vi "phd_pect.vi"() -> ()   [LabVIEW 2018]
uses:
  <vilib>/Instr/_visa.llb/VISA Configure Serial Port (Instr).vi
panel:
  out "str_ai_output":string caption="AI Output"
  out "num_sensor_sam_per_cycle":u32 caption="Samples/Cycle"
  in  "cbx_sensor_sam_rate":string(combo) caption="Sample Rate (Hz)"
  in  "num_pulse_samples":u32=3 caption="Samples" max=10000 step=100
  in  "Hidden Controls":T1(tab)
  out "baud rate":u32=115200
  out "timeout_default":u32=100
  out "termination char":u8
  out "timeout_for_small_data":u32=100
  out "CMD_ID_GET":string
  out "CMD_ID_RUN":string
  out "CMD_ID_NONE":string
  out "CMD_ID_SET":string
  out "CMD_RUN_NONE":string
  out "CMD_RUN_START":string
  out "CMD_RUN_STOP":string
  out "PG_PULSE_NONE":string
  out "PG_PULSE_SQUARE":string
  out "PG_PULSE_SINE":string
  out "RESPONSE_LEN":u32=32
  out "TIM_FREQ":u32
  out "has_response":bool=TRUE
  out "ADC_CONVERSION_CYCLES":dbl=8.5
  out "ADC_FREQ":u32=64000000
  out "ADC_SAMPLING_TIME":dbl[](array[numeric])
  out "ADC_CLOCK_PRESCALER":u32[](array[numeric])
  out "sam_rates":cluster{u32, u32, dbl}[](array[cluster])
  out "cbx_sensor_sam_rate_sel_idx":u32
  in  "num_senor_read_samples":u32=3 caption="Read Samples" max=10000 step=100
  in  "num_pulse_min_val":dbl=1.0 caption="Minimum Value (V)" min=0.0 max=1.0 step=0.1
  in  "num_pulse_dutyc":u32=100 caption="Duty Cycle (%)" max=100 step=10
  in  "num_pulse_max_val":dbl=3.3 caption="Maximum Value (V)" min=0.0 max=3.3 step=0.1
  out "write buffer":string
  in  "btn_get":bool
  in  "cbx_pulse_type":string(combo) caption="Type"
  in  "num_pulse_freq":u32=200 caption="Frequency (Hz)" max=2000 step=100
  in  "btn_set":bool
  in  "btn_start_stop":bool
  in  "VISA resource name":refnum<visa-resource-name>
  out "read buffer":string
  out "Waveform Graph":u8[](graph)
  # "Communication"
  # "Settings"
  # "Pulse"
  # "Sensor"
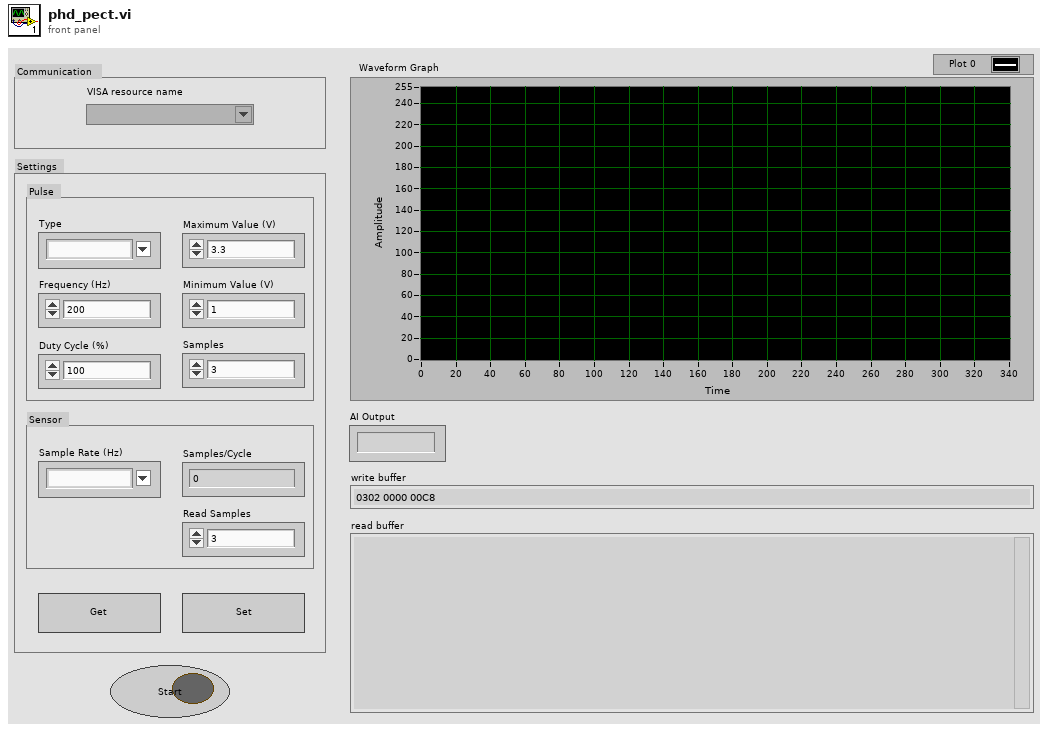
[diagram p1: front panel]
types:
  T1 = enum32{"Page 1", "Page 2", "Page 3", "Page 4", "Page 5"}
  T2 = enum8{"Enabled", "Disabled", "Disabled and Grayed Out"}
  T3 = enum16{"big-endian, network order", "native, host order", "little-endian"}
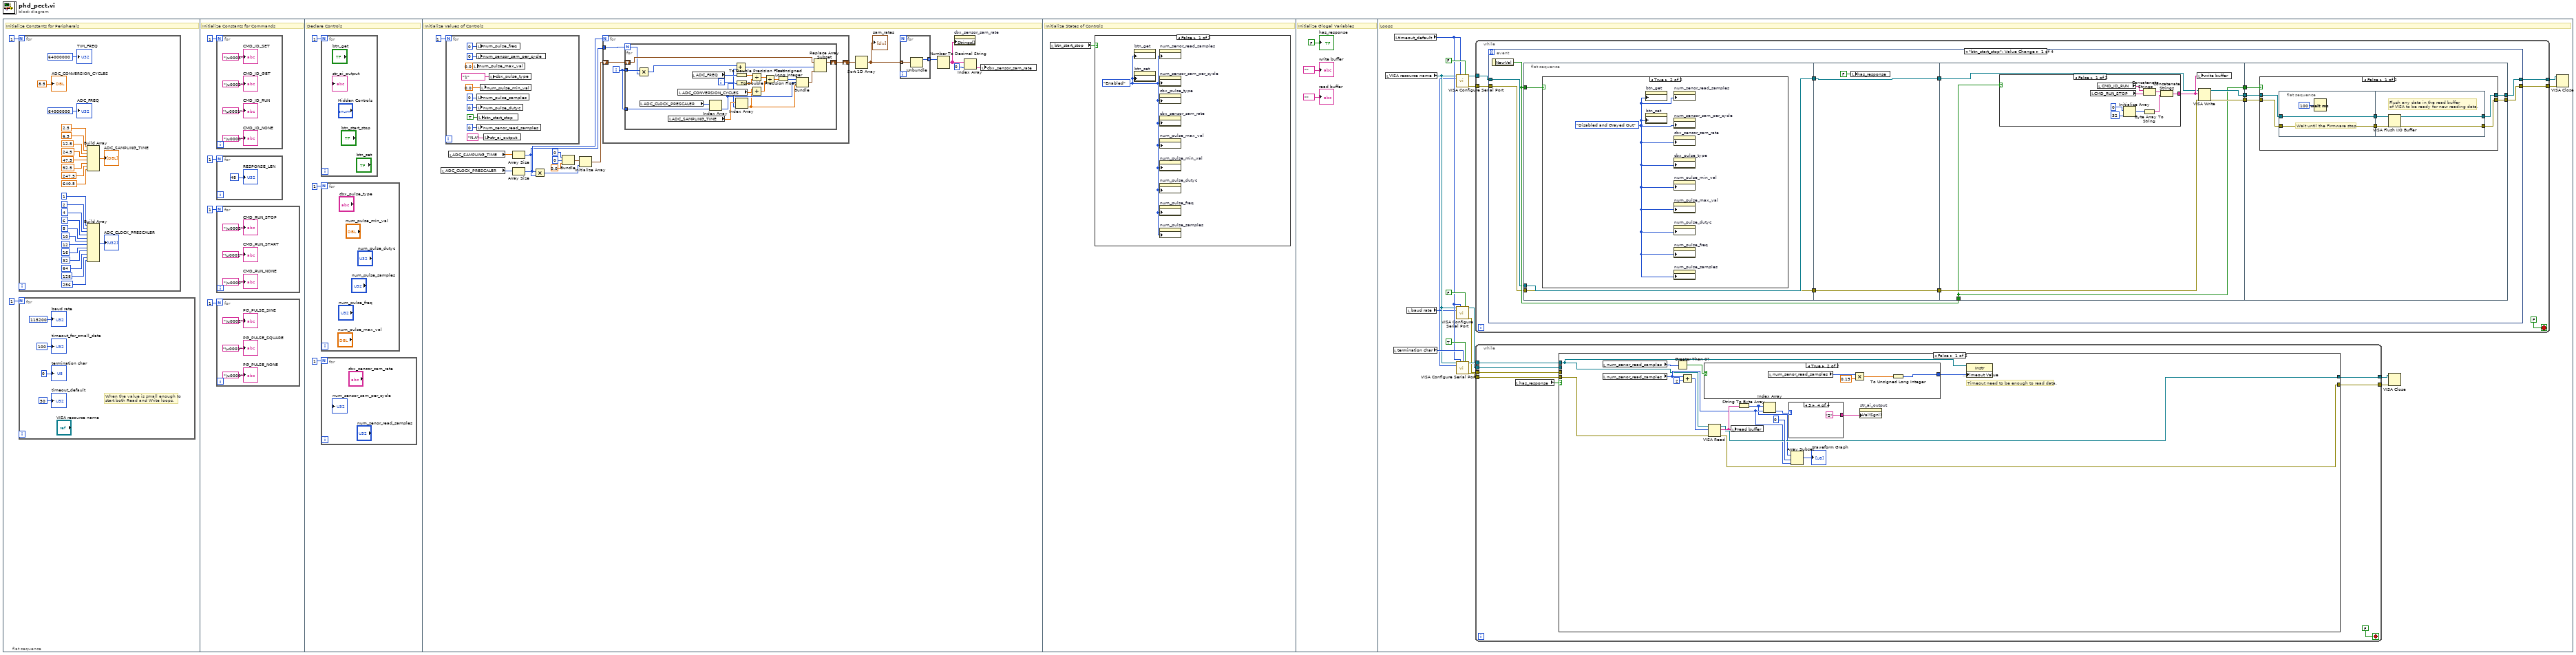
[diagram p0: block diagram]
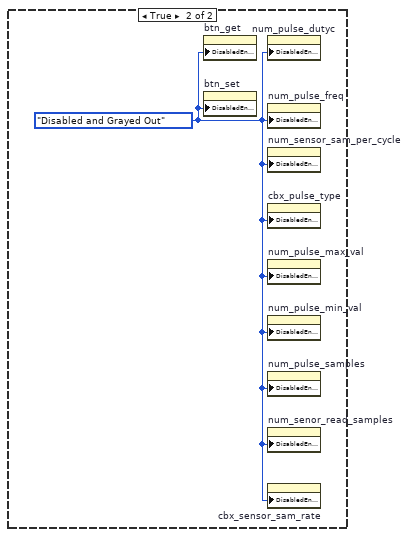
[diagram p2: hidden frame]
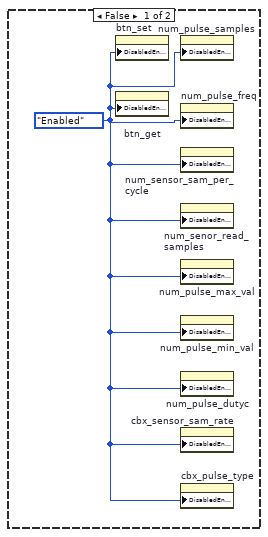
[diagram p3: hidden frame]
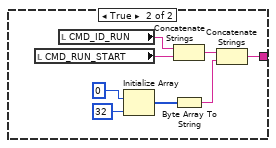
[diagram p4: hidden frame]
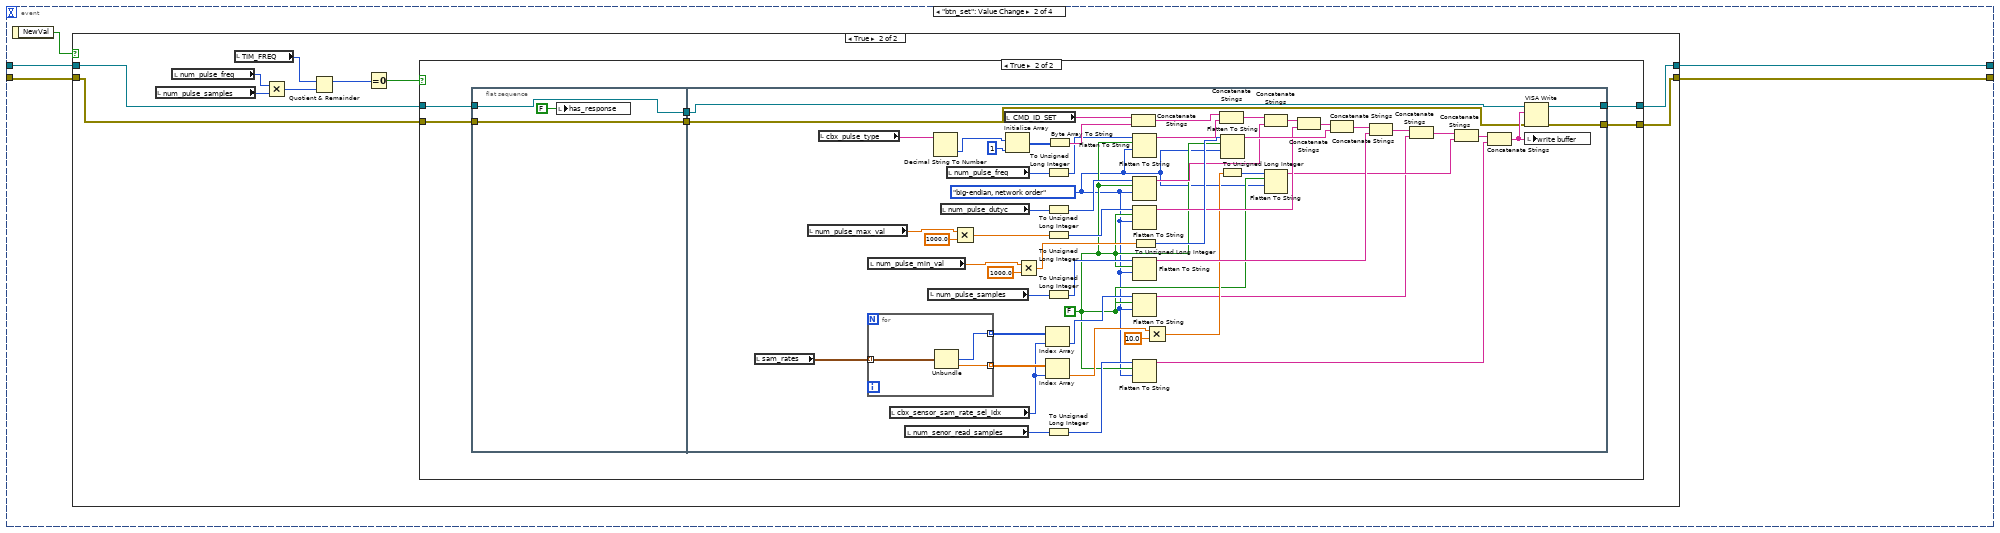
[diagram p6: hidden frame]
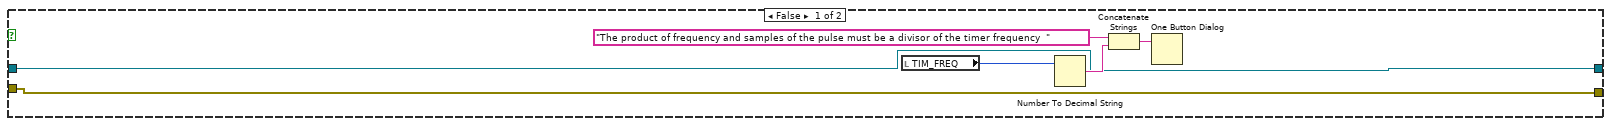
[diagram p8: hidden frame]
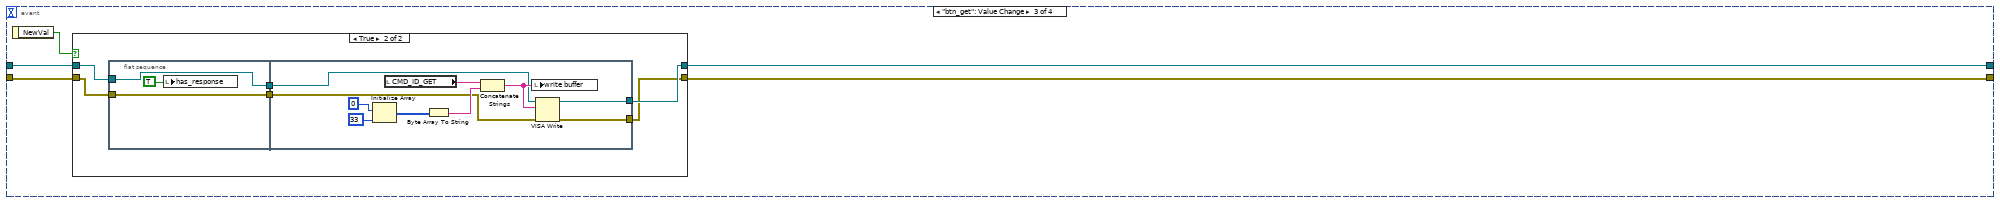
[diagram p9: hidden frame]
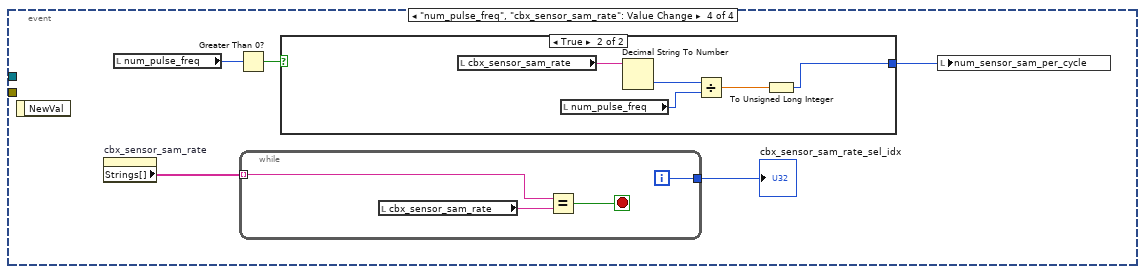
[diagram p11: hidden frame]
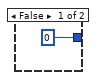
[diagram p12: hidden frame]
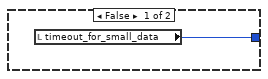
[diagram p13: hidden frame]
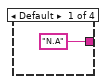
[diagram p14: hidden frame]
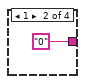
[diagram p15: hidden frame]
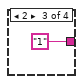
[diagram p16: hidden frame]
diagram:
  n1 = flat-sequence {
    frame #0 {
      # "Initialize Constants for Peripherals"
      n2 = for {
        N: 1 -> [_]
        n3 = Build Array(2.5 ("element"), 6.5 ("element"), 12.5 ("element"), 24.5 ("element"), 47.5 ("element"), 92.5 ("element"), 247.5 ("element"), 640.5 ("element")) -> (→"ADC_SAMPLING_TIME":dbl[])
        n4 = Build Array(u32 1 ("element"), u32 2 ("element"), u32 4 ("element"), u32 6 ("element"), u32 8 ("element"), u32 10 ("element"), u32 12 ("element"), u32 16 ("element"), u32 32 ("element"), u32 64 ("element"), u32 128 ("element"), u32 256 ("element")) -> (→"ADC_CLOCK_PRESCALER":u32[])
        "ADC_CONVERSION_CYCLES" <- 8.5
        "ADC_FREQ" <- 64000000
        "TIM_FREQ" <- 64000000
      }
      n5 = for {
        N: 1 -> [_]
        # "When the value is small enough to\nstart both Read and Write loops."
        "baud rate" <- u32 115200 ("baud rate (9600)")
        "timeout_default" <- u32 50 ("timeout (10sec)")
        "termination char" <- u8 0 ("termination char\n(0xA = '\\n' = LF)")
        "timeout_for_small_data" <- u32 100 ("timeout_default 2")
      }
    }
    frame #1 {
      # "Initialize Constants for Commands"
      n6 = for {
        N: 1 -> [_]
        "CMD_ID_NONE" <- "\u0000"
        "CMD_ID_RUN" <- "\u0001"
        "CMD_ID_GET" <- "\u0002"
        "CMD_ID_SET" <- "\u0003"
      }
      n7 = for {
        N: 1 -> [_]
        "RESPONSE_LEN" <- 48
      }
      n8 = for {
        N: 1 -> [_]
        "CMD_RUN_NONE" <- "\u0000"
        "CMD_RUN_START" <- "\u0001"
        "CMD_RUN_STOP" <- "\u0002"
      }
      n9 = for {
        N: 1 -> [_]
        "PG_PULSE_NONE" <- "\u0000"
        "PG_PULSE_SQUARE" <- "\u0001"
        "PG_PULSE_SINE" <- "\u0002"
      }
    }
    frame #2 {
      # "Declare Controls"
      n10 = for {
        N: 1 -> [_]
      }
      n11 = for {
        N: 1 -> [_]
      }
      n12 = for {
        N: 1 -> [_]
      }
    }
    frame #3 {
      # "Initialize Values of Controls"
      n13 = local read "ADC_CLOCK_PRESCALER"() -> (w60:u32[])
      n14 = for {
        N: 1 -> [_]
        n15 = local write "num_pulse_max_val"(0.0 ("num_pulse_amp")) -> ()
        n16 = local write "num_pulse_freq"(u32 0 ("num_pulse_freq")) -> ()
        n17 = local write "num_sensor_sam_per_cycle"(u32 0 ("num_sensor_sam_per_cycle")) -> ()
        n18 = local write "num_pulse_samples"(u32 0 ("num_pulse_samples")) -> ()
        n19 = local write "num_pulse_dutyc"(u32 0 ("num_pulse_dutyc")) -> ()
        n20 = local write "num_senor_read_samples"(u32 0 ("num_read_samples")) -> ()
        n21 = local write "btn_start_stop"(TRUE ("btn_start_stop")) -> ()
        n22 = local write "num_pulse_min_val"(0.0 ("num_pulse_amp_offset")) -> ()
        n23 = local write "str_ai_output"("N.A" ("str_ai_result")) -> ()
        n24 = local write "cbx_pulse_type"("1" ("cbx_pulse_type")) -> ()
      }
      n25 = local read "ADC_SAMPLING_TIME"() -> (w59:dbl[])
      n26 = Array Size(array=w59) -> (size(s)=w55:i32)
      n27 = Array Size(array=w60) -> (size(s)=w56:i32)
      n28 = Multiply(x=w56, y=w55) -> (x*y=w57:i32)
      n29 = Bundle(u32 0, u32 0, 0.0) -> (w61:cluster{u32, u32, dbl})  [unwired: 1 in]
      n30 = Initialize Array(w61, w57) -> (w54:cluster{u32, u32, dbl}[])
      n31 = for {
        N: w56 -> [_]
        tunnel: w55 -> [w72]
        shift-right: [w70] -> w58
        shift-left: w54 -> [w71]
        i -> [w69]
        n32 = for {
          N: w72 -> [w81]
          tunnel: w69 -> [w90]
          shift-right: [w78] -> w70
          shift-left: w71 -> [w84]
          tunnel: w69 -> [w82]
          i -> [w80]
          n33 = Multiply(x=w82, y=w81) -> (x*y=w83:i32)
          n34 = local read "ADC_CLOCK_PRESCALER"() -> (w91:u32[])
          n35 = local read "ADC_SAMPLING_TIME"() -> (w92:dbl[])
          n36 = local read "ADC_CONVERSION_CYCLES"() -> (w93:dbl)
          n37 = local read "ADC_FREQ"() -> (w86:u32)
          n38 = Index Array(array=w91, index=w90) -> (element=w74:u32)
          n39 = Add(x=w83, y=w80) -> (x+y=w79:i32)
          n40 = To Double Precision Float(number=w86) -> (double precision float=w85:dbl)
          n41 = To Double Precision Float(number=w74) -> (double precision float=w87:dbl)
          n42 = Index Array(array=w92, index=w80) -> (element=w73:dbl)
          n43 = Divide(x=w85, y=w87) -> (x/y=w89:dbl)
          n44 = Add(x=w93, y=w73) -> (x+y=w88:dbl)
          n45 = Divide(x=w89, y=w88) -> (x/y=w76:dbl)
          n46 = To Unsigned Long Integer(number=w76) -> (unsigned 32bit integer=w75:u32)
          n47 = Bundle(w75, "element"=w74, "element"=w73) -> (w77:cluster{u32, "element":u32, "element":dbl})  [unwired: 1 in]
          n48 = Replace Array Subset(array=w84, new element=w77, index=w79) -> (w78:cluster{u32, u32, dbl}[])
        }
      }
      n49 = Sort 1D Array(array=w58) -> (sorted array=w62:cluster{u32, u32, dbl}[])
      "sam_rates" <- w62
      n50 = for {
        tunnel: w62 -> [w68] mode=indexing
        tunnel: [w67] -> w63 mode=indexing
        n51 = Unbundle(w68) -> (w67:u32)  [unwired: 2 out]
      }
      n52 = Number To Decimal String(number=w63) -> (decimal integer string=w64:string[])  [unwired: 1 in]
      n53 = property on="cbx_sensor_sam_rate" class="CmbBox"("Strings[]"=w64) -> ()  [unwired: 2 in, 2 out]
      n54 = Index Array(array=w64, index=0) -> (element=w65:string)
      n55 = local write "cbx_sensor_sam_rate"(w65) -> ()
    }
    frame #4 {
      # "Initialize States of Controls"
      n56 = local read "btn_start_stop"() -> (w104:bool)
      n57 = case shown="False" w104 {
        frame False {
          w105 = T2."Enabled" ("Disabled")
          n58 = property on="btn_get" class="Bool (strict)"("DisabledEnum"=w105) -> ()  [unwired: 2 in, 2 out]
          n59 = property on="btn_set" class="Bool (strict)"("DisabledEnum"=w105) -> ()  [unwired: 2 in, 2 out]
          n60 = property on="num_senor_read_samples" class="DigNum (strict)"("DisabledEnum"=w105) -> ()  [unwired: 2 in, 2 out]
          n61 = property on="num_sensor_sam_per_cycle" class="DigNum (strict)"("DisabledEnum"=w105) -> ()  [unwired: 2 in, 2 out]
          n62 = property on="cbx_pulse_type" class="CmbBox"("DisabledEnum"=w105) -> ()  [unwired: 2 in, 2 out]
          n63 = property on="cbx_sensor_sam_rate" class="CmbBox"("DisabledEnum"=w105) -> ()  [unwired: 2 in, 2 out]
          n64 = property on="num_pulse_max_val" class="DigNum (strict)"("DisabledEnum"=w105) -> ()  [unwired: 2 in, 2 out]
          n65 = property on="num_pulse_min_val" class="DigNum (strict)"("DisabledEnum"=w105) -> ()  [unwired: 2 in, 2 out]
          n66 = property on="num_pulse_dutyc" class="DigNum (strict)"("DisabledEnum"=w105) -> ()  [unwired: 2 in, 2 out]
          n67 = property on="num_pulse_freq" class="DigNum (strict)"("DisabledEnum"=w105) -> ()  [unwired: 2 in, 2 out]
          n68 = property on="num_pulse_samples" class="DigNum (strict)"("DisabledEnum"=w105) -> ()  [unwired: 2 in, 2 out]
        }
        frame True {
          w106 = T2."Disabled and Grayed Out" ("Disabled")
          n69 = property on="btn_get" class="Bool (strict)"("DisabledEnum"=w106) -> ()  [unwired: 2 in, 2 out]
          n70 = property on="btn_set" class="Bool (strict)"("DisabledEnum"=w106) -> ()  [unwired: 2 in, 2 out]
          n71 = property on="num_pulse_dutyc" class="DigNum (strict)"("DisabledEnum"=w106) -> ()  [unwired: 2 in, 2 out]
          n72 = property on="num_pulse_freq" class="DigNum (strict)"("DisabledEnum"=w106) -> ()  [unwired: 2 in, 2 out]
          n73 = property on="num_sensor_sam_per_cycle" class="DigNum (strict)"("DisabledEnum"=w106) -> ()  [unwired: 2 in, 2 out]
          n74 = property on="cbx_pulse_type" class="CmbBox"("DisabledEnum"=w106) -> ()  [unwired: 2 in, 2 out]
          n75 = property on="num_pulse_max_val" class="DigNum (strict)"("DisabledEnum"=w106) -> ()  [unwired: 2 in, 2 out]
          n76 = property on="num_pulse_min_val" class="DigNum (strict)"("DisabledEnum"=w106) -> ()  [unwired: 2 in, 2 out]
          n77 = property on="num_pulse_samples" class="DigNum (strict)"("DisabledEnum"=w106) -> ()  [unwired: 2 in, 2 out]
          n78 = property on="num_senor_read_samples" class="DigNum (strict)"("DisabledEnum"=w106) -> ()  [unwired: 2 in, 2 out]
          n79 = property on="cbx_sensor_sam_rate" class="CmbBox"("DisabledEnum"=w106) -> ()  [unwired: 2 in, 2 out]
        }
      }
    }
    frame #5 {
      # "Initialize Glogal Variables"
      "write buffer" <- "" ("write buffer")
      "read buffer" <- "" ("read buffer")
      "has_response" <- FALSE
    }
    frame #6 {
      # "Loops"
      n80 = local read "VISA resource name"() -> (w111:refnum<visa-resource-name>)
      n81 = local read "termination char"() -> (w123:u8)
      n82 = local read "timeout_default"() -> (w112:u32)
      n83 = local read "baud rate"() -> (w110:u32)
      n84 = call-poly "VISA Configure Serial Port"("VISA resource name"=w111, "timeout (10sec)"=w112, "Enable Termination\nChar (T)"=FALSE ("Enable Termination\nChar (T)"), "baud rate (9600)"=w110) -> ("VISA resource name out"=w115:refnum<visa-resource-name>, "error out"=w114:errorcluster)  [unwired: 10 in]
      n85 = call-poly "VISA Configure Serial Port"("VISA resource name"=w111, "timeout (10sec)"=w112, "Enable Termination\nChar (T)"=FALSE ("Enable Termination\nChar (T)"), "baud rate (9600)"=w110) -> ("VISA resource name out"=w116:refnum<visa-resource-name>, "error out"=w117:errorcluster)  [unwired: 10 in]
      n86 = call-poly "VISA Configure Serial Port"("VISA resource name"=w111, "timeout (10sec)"=w112, "termination char\n(0xA = '\\n' = LF)"=w123, "Enable Termination\nChar (T)"=TRUE ("Enable Termination\nChar (T)"), "baud rate (9600)"=w110) -> ("VISA resource name out"=w124:refnum<visa-resource-name>, "error out"=w118:errorcluster)  [unwired: 9 in]
      n87 = while {
        tunnel: [w131] -> w120
        tunnel: [w130] -> w119
        tunnel: w115 -> [w127]
        tunnel: w114 -> [w128]
        stop <- FALSE stop-if-true
        n88 = event shown="[0] \"btn_start_stop\": Value Change" {
          selector: _ -> [_ _ _ _]
          dyn-events: _ -> [_ _ _ _]
          timeout: _ -> [_ _ _ _]
          tunnel: [w133 w197 w284 _] -> w131
          tunnel: [w132 w196 w283 _] -> w130
          tunnel: w128 -> [w137 w194 w286 _]
          tunnel: w127 -> [w138 w195 w285 _]
          event "btn_start_stop": Value Change {
            n89 = event-data() -> ("NewVal"=w143:bool)  [unwired: 1 in]
            n90 = flat-sequence {
              tunnel: w143 -> [w146]
              tunnel: w138 -> [w145]
              tunnel: [w145] -> w142
              tunnel: w137 -> [w144]
              tunnel: [w144] -> w140
              tunnel: w142 -> [w150]
              tunnel: [w150] -> w141
              tunnel: w140 -> [w149]
              tunnel: [w149] -> w139
              tunnel: w143 -> [w152]
              tunnel: w141 -> [w156]
              tunnel: w139 -> [w155]
              tunnel: [w154] -> w136
              tunnel: [w153] -> w135
              tunnel: [w152] -> w134
              tunnel: w136 -> [w177]
              tunnel: w135 -> [w176]
              tunnel: w134 -> [w178]
              tunnel: [w175] -> w133
              tunnel: [w174] -> w132
              frame #0 {
                n91 = case shown="True" w146 {
                  frame False {
                    w147 = T2."Enabled" ("Disabled")
                    n92 = property on="btn_set" class="Bool (strict)"("DisabledEnum"=w147) -> ()  [unwired: 2 in, 2 out]
                    n93 = property on="btn_get" class="Bool (strict)"("DisabledEnum"=w147) -> ()  [unwired: 2 in, 2 out]
                    n94 = property on="num_pulse_samples" class="DigNum (strict)"("DisabledEnum"=w147) -> ()  [unwired: 2 in, 2 out]
                    n95 = property on="num_pulse_freq" class="DigNum (strict)"("DisabledEnum"=w147) -> ()  [unwired: 2 in, 2 out]
                    n96 = property on="num_sensor_sam_per_cycle" class="DigNum (strict)"("DisabledEnum"=w147) -> ()  [unwired: 2 in, 2 out]
                    n97 = property on="num_senor_read_samples" class="DigNum (strict)"("DisabledEnum"=w147) -> ()  [unwired: 2 in, 2 out]
                    n98 = property on="num_pulse_max_val" class="DigNum (strict)"("DisabledEnum"=w147) -> ()  [unwired: 2 in, 2 out]
                    n99 = property on="num_pulse_min_val" class="DigNum (strict)"("DisabledEnum"=w147) -> ()  [unwired: 2 in, 2 out]
                    n100 = property on="num_pulse_dutyc" class="DigNum (strict)"("DisabledEnum"=w147) -> ()  [unwired: 2 in, 2 out]
                    n101 = property on="cbx_sensor_sam_rate" class="CmbBox"("DisabledEnum"=w147) -> ()  [unwired: 2 in, 2 out]
                    n102 = property on="cbx_pulse_type" class="CmbBox"("DisabledEnum"=w147) -> ()  [unwired: 2 in, 2 out]
                  }
                  frame True {
                    w148 = T2."Disabled and Grayed Out" ("Disabled")
                    n103 = property on="btn_get" class="Bool (strict)"("DisabledEnum"=w148) -> ()  [unwired: 2 in, 2 out]
                    n104 = property on="btn_set" class="Bool (strict)"("DisabledEnum"=w148) -> ()  [unwired: 2 in, 2 out]
                    n105 = property on="num_senor_read_samples" class="DigNum (strict)"("DisabledEnum"=w148) -> ()  [unwired: 2 in, 2 out]
                    n106 = property on="num_sensor_sam_per_cycle" class="DigNum (strict)"("DisabledEnum"=w148) -> ()  [unwired: 2 in, 2 out]
                    n107 = property on="cbx_sensor_sam_rate" class="CmbBox"("DisabledEnum"=w148) -> ()  [unwired: 2 in, 2 out]
                    n108 = property on="cbx_pulse_type" class="CmbBox"("DisabledEnum"=w148) -> ()  [unwired: 2 in, 2 out]
                    n109 = property on="num_pulse_min_val" class="DigNum (strict)"("DisabledEnum"=w148) -> ()  [unwired: 2 in, 2 out]
                    n110 = property on="num_pulse_max_val" class="DigNum (strict)"("DisabledEnum"=w148) -> ()  [unwired: 2 in, 2 out]
                    n111 = property on="num_pulse_dutyc" class="DigNum (strict)"("DisabledEnum"=w148) -> ()  [unwired: 2 in, 2 out]
                    n112 = property on="num_pulse_freq" class="DigNum (strict)"("DisabledEnum"=w148) -> ()  [unwired: 2 in, 2 out]
                    n113 = property on="num_pulse_samples" class="DigNum (strict)"("DisabledEnum"=w148) -> ()  [unwired: 2 in, 2 out]
                  }
                }
              }
              frame #1 {
                n114 = local write "has_response"(FALSE ("IS_RESPONSE")) -> ()
              }
              frame #2 {
                n115 = case shown="False" w152 {
                  tunnel: [w162 w170] -> w157
                  frame False {
                    n116 = local read "CMD_RUN_STOP"() -> (w163:string)
                    n117 = local read "CMD_ID_RUN"() -> (w164:string)
                    n118 = Initialize Array(u8 0 ("element"), 32 ("dimension size")) -> (w159:u8[])
                    n119 = Concatenate Strings(w164, w163) -> (w165:string)
                    n120 = Byte Array To String(unsigned byte array=w159) -> (string=w158:string)
                    n121 = Concatenate Strings(w165, w158) -> (w162:string)
                  }
                  frame True {
                    n122 = local read "CMD_RUN_START"() -> (w172:string)
                    n123 = local read "CMD_ID_RUN"() -> (w173:string)
                    n124 = Initialize Array(u8 0 ("element"), 32 ("dimension size")) -> (w167:u8[])
                    n125 = Concatenate Strings(w173, w172) -> (w171:string)
                    n126 = Byte Array To String(unsigned byte array=w167) -> (string=w166:string)
                    n127 = Concatenate Strings(w171, w166) -> (w170:string)
                  }
                }
                n128 = local write "write buffer"(w157) -> ()
                n129 = VISA Write(VISA resource name=w156, write buffer=w157, error in (no error)=w155) -> (VISA resource name out=w154:refnum<visa-resource-name>, error out=w153:errorcluster)  [unwired: 1 out]
              }
              frame #3 {
                n130 = case shown="False" w178 {
                  tunnel: w177 -> [w184 w193]
                  tunnel: w176 -> [w182 w192]
                  tunnel: [w180 w193] -> w175
                  tunnel: [w179 w192] -> w174
                  frame False {
                    n131 = flat-sequence {
                      tunnel: w184 -> [w186]
                      tunnel: [w186] -> w183
                      tunnel: w182 -> [w185]
                      tunnel: [w185] -> w181
                      tunnel: w183 -> [w191]
                      tunnel: w181 -> [w190]
                      tunnel: [w189] -> w180
                      tunnel: [w188] -> w179
                      frame #0 {
                        # "Wait until the Firmware stop"
                        n132 = Wait (ms)(milliseconds to wait=u32 100) -> ()  [unwired: 1 out]
                      }
                      frame #1 {
                        # "Flush any data in the read buffer\nof VISA to be ready for new reading data."
                        n133 = VISA Flush I/O Buffer(VISA resource name=w191, error in (no error)=w190) -> (VISA resource name out=w189:refnum<visa-resource-name>, error out=w188:errorcluster)  [unwired: 1 in]
                      }
                    }
                  }
                  frame True {
                  }
                }
              }
            }
          }
          event "btn_set": Value Change {
            n134 = event-data() -> ("NewVal"=w198:bool)  [unwired: 1 in]
            n135 = case shown="True" w198 {
              tunnel: w195 -> [w200 w204]
              tunnel: w194 -> [w199 w203]
              tunnel: [w200 w202] -> w197
              tunnel: [w199 w201] -> w196
              frame False {
              }
              frame True {
                n136 = local read "num_pulse_samples"() -> (w205:u32)
                n137 = local read "num_pulse_freq"() -> (w207:u32)
                n138 = local read "TIM_FREQ"() -> (w208:u32)
                n139 = Multiply(x=w207, y=w205) -> (x*y=w206:u32)
                n140 = Quotient & Remainder(x=w208, y=w206) -> (x-y*floor(x/y)=w210:u32)  [unwired: 1 out]
                n141 = Equal To 0?(x=w210) -> (x = 0?=w209:bool)
                n142 = case shown="True" w209 {
                  tunnel: w204 -> [w212 w222]
                  tunnel: w203 -> [w211 w220]
                  tunnel: [w212 w218] -> w202
                  tunnel: [w211 w217] -> w201
                  frame False {
                    n143 = local read "TIM_FREQ"() -> (w213:u32)
                    n144 = Number To Decimal String(number=w213) -> (decimal integer string=w215:string)  [unwired: 1 in]
                    n145 = Concatenate Strings("The product of frequency and samples of the pulse must be a divisor of the timer frequency  " ("string"), w215) -> (w214:string)
                    n146 = One Button Dialog(message=w214) -> ()  [unwired: 1 in, 1 out]
                  }
                  frame True {
                    n147 = flat-sequence {
                      tunnel: w222 -> [w224]
                      tunnel: [w224] -> w221
                      tunnel: w220 -> [w223]
                      tunnel: [w223] -> w219
                      tunnel: w221 -> [w229]
                      tunnel: w219 -> [w228]
                      tunnel: [w227] -> w218
                      tunnel: [w226] -> w217
                      frame #0 {
                        n148 = local write "has_response"(FALSE ("IS_RESPONSE")) -> ()
                      }
                      frame #1 {
                        w237 = FALSE ("prepend array or string size? (T)")
                        w236 = T3."big-endian, network order" ("byte order (0:big-endian, network order)")
                        n149 = local read "sam_rates"() -> (w245:cluster{u32, u32, dbl}[])
                        n150 = local read "num_pulse_max_val"() -> (w274:dbl)
                        n151 = local read "cbx_pulse_type"() -> (w276:string)
                        n152 = for {
                          tunnel: w245 -> [w282] mode=indexing
                          tunnel: [w281] -> w244 mode=indexing
                          tunnel: [w280] -> w243 mode=indexing
                          n153 = Unbundle(w282) -> (w280:u32, w281:dbl)  [unwired: 1 out]
                        }
                        n154 = local read "num_pulse_min_val"() -> (w272:dbl)
                        n155 = local read "cbx_sensor_sam_rate_sel_idx"() -> (w230:u32)
                        n156 = local read "num_senor_read_samples"() -> (w255:u32)
                        n157 = local read "num_pulse_samples"() -> (w250:u32)
                        n158 = Decimal String To Number(string=w276) -> (number=w277:i32)  [unwired: 2 in, 1 out]
                        n159 = local read "num_pulse_dutyc"() -> (w252:u32)
                        n160 = local read "num_pulse_freq"() -> (w253:u32)
                        n161 = Multiply(x=w274, y=1000.0) -> (x*y=w273:dbl)
                        n162 = local read "CMD_ID_SET"() -> (w262:string)
                        n163 = Initialize Array(w277, 1 ("dimension size")) -> (w278:i32[])
                        n164 = Multiply(x=w272, y=1000.0) -> (x*y=w270:dbl)
                        n165 = Index Array(array=w243, index=w230) -> (element=w242:u32)
                        n166 = Index Array(array=w244, index=w230) -> (element=w241:dbl)
                        n167 = To Unsigned Long Integer(number=w253) -> (unsigned 32bit integer=w254:u32)
                        n168 = To Unsigned Long Integer(number=w252) -> (unsigned 32bit integer=w251:u32)
                        n169 = To Unsigned Long Integer(number=w273) -> (unsigned 32bit integer=w275:u32)
                        n170 = To Unsigned Long Integer(number=w250) -> (unsigned 32bit integer=w249:u32)
                        n171 = To Unsigned Long Integer(number=w255) -> (unsigned 32bit integer=w246:u32)
                        n172 = Byte Array To String(unsigned byte array=w278) -> (string=w279:string)
                        n173 = Concatenate Strings(w262, w279) -> (w264:string)
                        n174 = Flatten To String(anything=w254, prepend array or string size? (T)=w237, byte order (0:big-endian, network order)=w236) -> (data string=w263:string)  [unwired: 1 in, 2 out]
                        n175 = Flatten To String(anything=w251, prepend array or string size? (T)=w237, byte order (0:big-endian, network order)=w236) -> (data string=w267:string)  [unwired: 1 in, 2 out]
                        n176 = Flatten To String(anything=w275, prepend array or string size? (T)=w237, byte order (0:big-endian, network order)=w236) -> (data string=w261:string)  [unwired: 1 in, 2 out]
                        n177 = Flatten To String(anything=w249, prepend array or string size? (T)=w237, byte order (0:big-endian, network order)=w236) -> (data string=w256:string)  [unwired: 1 in, 2 out]
                        n178 = Flatten To String(anything=w242, prepend array or string size? (T)=w237, byte order (0:big-endian, network order)=w236) -> (data string=w233:string)  [unwired: 1 in, 2 out]
                        n179 = Flatten To String(anything=w246, prepend array or string size? (T)=w237, byte order (0:big-endian, network order)=w236) -> (data string=w248:string)  [unwired: 1 in, 2 out]
                        n180 = To Unsigned Long Integer(number=w270) -> (unsigned 32bit integer=w271:u32)
                        n181 = Multiply(x=w241, y=10.0) -> (x*y=w239:dbl)
                        n182 = Concatenate Strings(w264, w263) -> (w265:string)
                        n183 = Flatten To String(anything=w271, prepend array or string size? (T)=w237, byte order (0:big-endian, network order)=w236) -> (data string=w269:string)  [unwired: 1 in, 2 out]
                        n184 = To Unsigned Long Integer(number=w239) -> (unsigned 32bit integer=w238:u32)
                        n185 = Concatenate Strings(w265, w267) -> (w266:string)
                        n186 = Flatten To String(anything=w238, prepend array or string size? (T)=w237, byte order (0:big-endian, network order)=w236) -> (data string=w234:string)  [unwired: 1 in, 2 out]
                        n187 = Concatenate Strings(w266, w261) -> (w268:string)
                        n188 = Concatenate Strings(w268, w269) -> (w257:string)
                        n189 = Concatenate Strings(w257, w256) -> (w232:string)
                        n190 = Concatenate Strings(w232, w233) -> (w235:string)
                        n191 = Concatenate Strings(w235, w234) -> (w231:string)
                        n192 = Concatenate Strings(w231, w248) -> (w247:string)
                        n193 = VISA Write(VISA resource name=w229, write buffer=w247, error in (no error)=w228) -> (VISA resource name out=w227:refnum<visa-resource-name>, error out=w226:errorcluster)  [unwired: 1 out]
                        n194 = local write "write buffer"(w247) -> ()
                      }
                    }
                  }
                }
              }
            }
          }
          event "btn_get": Value Change {
            n195 = event-data() -> ("NewVal"=w287:bool)  [unwired: 1 in]
            n196 = case shown="True" w287 {
              tunnel: w285 -> [w289 w295]
              tunnel: w286 -> [w288 w293]
              tunnel: [w289 w291] -> w284
              tunnel: [w288 w290] -> w283
              frame False {
              }
              frame True {
                n197 = flat-sequence {
                  tunnel: w295 -> [w297]
                  tunnel: [w297] -> w294
                  tunnel: w293 -> [w296]
                  tunnel: [w296] -> w292
                  tunnel: w294 -> [w302]
                  tunnel: w292 -> [w301]
                  tunnel: [w300] -> w291
                  tunnel: [w299] -> w290
                  frame #0 {
                    n198 = local write "has_response"(TRUE ("IS_RESPONSE")) -> ()
                  }
                  frame #1 {
                    n199 = Initialize Array(u8 0 ("element"), 33 ("dimension size")) -> (w304:u8[])
                    n200 = local read "CMD_ID_GET"() -> (w308:string)
                    n201 = Byte Array To String(unsigned byte array=w304) -> (string=w303:string)
                    n202 = Concatenate Strings(w308, w303) -> (w307:string)
                    n203 = local write "write buffer"(w307) -> ()
                    n204 = VISA Write(VISA resource name=w302, write buffer=w307, error in (no error)=w301) -> (VISA resource name out=w300:refnum<visa-resource-name>, error out=w299:errorcluster)  [unwired: 1 out]
                  }
                }
              }
            }
          }
          event "num_pulse_freq", "cbx_sensor_sam_rate": Value Change {
            n205 = event-data() -> ()  [unwired: 1 in, 1 out]
            n206 = property on="cbx_sensor_sam_rate" class="CmbBox"() -> ("Strings[]"=w312:string[])  [unwired: 2 in, 2 out]
            n207 = local read "num_pulse_freq"() -> (w309:u32)
            n208 = Greater Than 0?(x=w309) -> (x > 0?=w310:bool)
            n209 = while {
              tunnel: w312 -> [w317] mode=indexing
              tunnel: [w314] -> w313
              i -> [w314]
              stop <- w315 stop-if-true
              n210 = local read "cbx_sensor_sam_rate"() -> (w316:string)
              n211 = Equal?(x=w317, y=w316) -> (x = y?=w315:bool)
            }
            "cbx_sensor_sam_rate_sel_idx" <- w313
            n212 = case shown="True" w310 {
              tunnel: [0 w323] -> w311
              frame False {
              }
              frame True {
                n213 = local read "cbx_sensor_sam_rate"() -> (w319:string)
                n214 = local read "num_pulse_freq"() -> (w321:u32)
                n215 = Decimal String To Number(string=w319) -> (number=w320:i32)  [unwired: 2 in, 1 out]
                n216 = Divide(x=w320, y=w321) -> (x/y=w322:dbl)
                n217 = To Unsigned Long Integer(number=w322) -> (unsigned 32bit integer=w323:u32)
              }
            }
            n218 = local write "num_sensor_sam_per_cycle"(w311) -> ()
          }
        }
      }
      n219 = while {
        tunnel: w124 -> [w329]
        tunnel: w118 -> [w330]
        tunnel: [w328] -> w125
        tunnel: [w327] -> w126
        tunnel: w116 -> [w326]
        tunnel: w117 -> [w325]
        stop <- FALSE stop-if-true
        n220 = local read "has_response"() -> (w331:bool)
        n221 = case shown="False" w331 {
          tunnel: w330 -> [w344 _]
          tunnel: w329 -> [w333 _]
          tunnel: [w343 w359] -> w327
          tunnel: [w342 w361] -> w328
          tunnel: w326 -> [_ w357]
          tunnel: w325 -> [_ w362]
          frame False {
            # "Timeout need to be enough to read data."
            n222 = local read "num_senor_read_samples"() -> (w335:u32)
            n223 = local read "num_senor_read_samples"() -> (w339:u32)
            n224 = Greater Than 0?(x=w335) -> (x > 0?=w334:bool)
            n225 = Add(x=w339, y=u32 2) -> (x+y=w340:u32)
            n226 = case shown="True" w334 {
              tunnel: [w348 w349] -> w332
              frame False {
                n227 = local read "timeout_for_small_data"() -> (w348:u32)
              }
              frame True {
                n228 = local read "num_senor_read_samples"() -> (w352:u32)
                n229 = Multiply(x=w352, y=0.15) -> (x*y=w350:dbl)
                n230 = To Unsigned Long Integer(number=w350) -> (unsigned 32bit integer=w349:u32)
              }
            }
            n231 = VISA Read(VISA resource name=w333, byte count=w340, error in (no error)=w344) -> (VISA resource name out=w342:refnum<visa-resource-name>, read buffer=w347:string, error out=w343:errorcluster)  [unwired: 1 out]
            n232 = local write "read buffer"(w347) -> ()
            n233 = String To Byte Array(string=w347) -> (unsigned byte array=w338:u8[])
            n234 = Index Array(array=w338, index=w339) -> (element=w337:u8)
            n235 = case shown="3" w337 {
              tunnel: ["N.A" "0" "1" "2"] -> w336
              frame Default {
              }
              frame 1 {
              }
              frame 2 {
              }
              frame 3 {
              }
            }
            n236 = Array Subset(array=w338, index=0, length=w339) -> (→"Waveform Graph":u8[])
            n237 = property on="str_ai_output" class="Str"("Val(Sgnl)"=w336) -> ()  [unwired: 2 in, 2 out]
            n238 = property class="Instr"(reference=w333, "General Settings:Timeout Value"=w332) -> ()  [unwired: 1 in, 2 out]
          }
          frame True {
            n239 = flat-sequence {
              tunnel: w357 -> [w370]
              tunnel: w362 -> [w369]
              tunnel: [w368] -> w360
              tunnel: [w367] -> w358
              tunnel: [w435] -> w361
              tunnel: w360 -> [w435]
              tunnel: [w434] -> w359
              tunnel: w358 -> [w434]
              frame #0 {
                n240 = local read "RESPONSE_LEN"() -> (w373:u32)
                n241 = local read "CMD_ID_GET"() -> (w364:string)
                n242 = VISA Read(VISA resource name=w370, byte count=w373, error in (no error)=w369) -> (VISA resource name out=w368:refnum<visa-resource-name>, read buffer=w371:string, error out=w367:errorcluster)  [unwired: 1 out]
                n243 = local write "read buffer"(w371) -> ()
                n244 = String To Byte Array(string=w364) -> (unsigned byte array=w366:u8[])
                n245 = String To Byte Array(string=w371) -> (unsigned byte array=w376:u8[])
                n246 = Index Array(array=w376, index=0) -> (element=w374:u8)
                n247 = Index Array(array=w366, index=0) -> (element=w363:u8)
                n248 = Equal?(x=w374, y=w363) -> (x = y?=w375:bool)
                n249 = case shown="True" w375 {
                  tunnel: w376 -> [_ w433]
                  tunnel: w371 -> [_ w393]
                  frame False {
                  }
                  frame True {
                    w392 = FALSE ("data includes array or string size? (T)")
                    w391 = T3."big-endian, network order" ("byte order (0:big-endian, network order)")
                    n250 = Index Array(array=w433, index=1) -> (element=w415:u8)
                    n251 = String Subset(string=w393, offset (0)=18, length (rest)=4 ("length (rest)")) -> (substring=w413:string)
                    n252 = String Subset(string=w393, offset (0)=14, length (rest)=4 ("length (rest)")) -> (substring=w416:string)
                    n253 = String Subset(string=w393, offset (0)=10, length (rest)=4 ("length (rest)")) -> (substring=w423:string)
                    n254 = String Subset(string=w393, offset (0)=30, length (rest)=4 ("length (rest)")) -> (substring=w410:string)
                    n255 = String Subset(string=w393, offset (0)=22, length (rest)=4 ("length (rest)")) -> (substring=w398:string)
                    n256 = String Subset(string=w393, offset (0)=26, length (rest)=4 ("length (rest)")) -> (substring=w395:string)
                    n257 = Number To Decimal String(number=w415) -> (decimal integer string=w401:string)  [unwired: 1 in]
                    n258 = property on="cbx_pulse_type" class="CmbBox"("Val(Sgnl)"=w401) -> ()  [unwired: 2 in, 2 out]
                    n259 = String Subset(string=w393, offset (0)=2, length (rest)=4 ("length (rest)")) -> (substring=w425:string)
                    n260 = String Subset(string=w393, offset (0)=6, length (rest)=4 ("length (rest)")) -> (substring=w424:string)
                    n261 = To Unsigned Long Integer(number=u32 0) -> (unsigned 32bit integer=w390:u32)
                    n262 = local read "ADC_FREQ"() -> (w387:u32)
                    n263 = Unflatten From String(type=w390, binary string=w413, data includes array or string size? (T)=w392, byte order (0:big-endian, network order)=w391) -> (value=w402:u32)  [unwired: 1 in, 2 out]
                    n264 = Unflatten From String(type=w390, binary string=w416, data includes array or string size? (T)=w392, byte order (0:big-endian, network order)=w391) -> (value=w420:u32)  [unwired: 1 in, 2 out]
                    n265 = Unflatten From String(type=w390, binary string=w410, data includes array or string size? (T)=w392, byte order (0:big-endian, network order)=w391) -> (value=w404:u32)  [unwired: 1 in, 2 out]
                    n266 = Unflatten From String(type=w390, binary string=w398, data includes array or string size? (T)=w392, byte order (0:big-endian, network order)=w391) -> (value=w384:u32)  [unwired: 1 in, 2 out]
                    n267 = Unflatten From String(type=w390, binary string=w395, data includes array or string size? (T)=w392, byte order (0:big-endian, network order)=w391) -> (value=w389:u32)  [unwired: 1 in, 2 out]
                    n268 = Unflatten From String(type=w390, binary string=w423, data includes array or string size? (T)=w392, byte order (0:big-endian, network order)=w391) -> (value=w422:u32)  [unwired: 1 in, 2 out]
                    n269 = Unflatten From String(type=w390, binary string=w425, data includes array or string size? (T)=w392, byte order (0:big-endian, network order)=w391) -> (value=w407:u32)  [unwired: 1 in, 2 out]
                    n270 = Unflatten From String(type=w390, binary string=w424, data includes array or string size? (T)=w392, byte order (0:big-endian, network order)=w391) -> (value=w406:u32)  [unwired: 1 in, 2 out]
                    n271 = local read "ADC_CONVERSION_CYCLES"() -> (w383:dbl)
                    n272 = property on="num_pulse_samples" class="DigNum (strict)"("Val(Sgnl)"=w402) -> ()  [unwired: 2 in, 2 out]
                    n273 = property on="num_senor_read_samples" class="DigNum (strict)"("Val(Sgnl)"=w404) -> ()  [unwired: 2 in, 2 out]
                    n274 = property on="num_pulse_freq" class="DigNum (strict)"("Val(Sgnl)"=w407) -> ()  [unwired: 2 in, 2 out]
                    n275 = property on="num_pulse_dutyc" class="DigNum (strict)"("Val(Sgnl)"=w406) -> ()  [unwired: 2 in, 2 out]
                    n276 = To Double Precision Float(number=w387) -> (double precision float=w386:dbl)
                    n277 = To Double Precision Float(number=w384) -> (double precision float=w385:dbl)
                    n278 = To Double Precision Float(number=w389) -> (double precision float=w394:dbl)
                    n279 = Divide(x=w420, y=1000.0) -> (x/y=w403:dbl)
                    n280 = Divide(x=w422, y=1000.0) -> (x/y=w405:dbl)
                    n281 = Divide(x=w386, y=w385) -> (x/y=w381:dbl)
                    n282 = Divide(x=w394, y=10.0) -> (x/y=w382:dbl)
                    n283 = property on="num_pulse_min_val" class="DigNum (strict)"("Val(Sgnl)"=w403) -> ()  [unwired: 2 in, 2 out]
                    n284 = property on="num_pulse_max_val" class="DigNum (strict)"("Val(Sgnl)"=w405) -> ()  [unwired: 2 in, 2 out]
                    n285 = Add(x=w383, y=w382) -> (x+y=w380:dbl)
                    n286 = Divide(x=w381, y=w380) -> (x/y=w379:dbl)
                    n287 = To Unsigned Long Integer(number=w379) -> (unsigned 32bit integer=w378:u32)
                    n288 = Number To Decimal String(number=w378) -> (decimal integer string=w377:string)  [unwired: 1 in]
                    n289 = property on="cbx_sensor_sam_rate" class="CmbBox"("Val(Sgnl)"=w377) -> ()  [unwired: 2 in, 2 out]
                  }
                }
              }
              frame #1 {
                n290 = local write "has_response"(FALSE ("IS_RESPONSE")) -> ()
              }
            }
          }
        }
      }
      n291 = VISA Close(VISA resource name=w125, error in (no error)=w126) -> ()  [unwired: 1 out]
      n292 = VISA Close(VISA resource name=w120, error in (no error)=w119) -> ()  [unwired: 1 out]
    }
  }
